vi "Sensors Begin.vi"   [LabVIEW 2013]
uses:
  <vilib>/Rock Robotics/SystemInterfaces/AI/FPGA_AIChannel.ctl
  <vilib>/Rock Robotics/SystemInterfaces/Typedef/FPGA_TypedefAnalogModule.ctl
types:
  T1 = typedef "FPGA_AIChannel.ctl" = enum8{"AI 1", "AI 2", "AI 3", "AI 4", "AI 5", "AI 6", "AI 7", "AI 8", "Invalid"}
  T2 = typedef "FPGA_TypedefAnalogModule.ctl" = enum16{"Analog Module 1", "Analog Module 2"}
  T3 = typedef "WPI_AnalogChannelDevRef.ctl" = cluster{"DevStatus":errorcluster, "Analog Module":T2, "Analog Channel":T1}
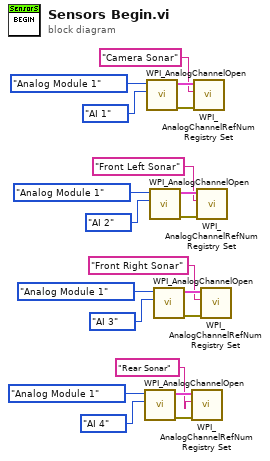
[diagram p0: block diagram]
diagram:
  n1 = call <vilib>:"WPI_AnalogChannelOpen.vi"("Analog Channel"=FPGA_AIChannel."AI 4", "Analog Module (Module 1)"=FPGA_TypedefAnalogModule."Analog Module 1") -> ("error out"=w5:errorcluster, "AIDeviceRef"=w4:T3)  [unwired: 8 in]
  n2 = call <vilib>:"WPI_AnalogChannelOpen.vi"("Analog Channel"=FPGA_AIChannel."AI 1", "Analog Module (Module 1)"=FPGA_TypedefAnalogModule."Analog Module 1") -> ("error out"=w19:errorcluster, "AIDeviceRef"=w20:T3)  [unwired: 8 in]
  n3 = call <vilib>:"WPI_AnalogChannelOpen.vi"("Analog Channel"=FPGA_AIChannel."AI 2", "Analog Module (Module 1)"=FPGA_TypedefAnalogModule."Analog Module 1") -> ("error out"=w13:errorcluster, "AIDeviceRef"=w12:T3)  [unwired: 8 in]
  n4 = call <vilib>:"WPI_AnalogChannelOpen.vi"("Analog Channel"=FPGA_AIChannel."AI 3", "Analog Module (Module 1)"=FPGA_TypedefAnalogModule."Analog Module 1") -> ("error out"=w10:errorcluster, "AIDeviceRef"=w11:T3)  [unwired: 8 in]
  n5 = call <vilib>:"WPI_AnalogChannelRefNum Registry Set.vi"("error in (no error)"=w5, "refnum name"="Rear Sonar", "AIDeviceRef"=w4) -> ()  [unwired: 7 in, 2 out]
  n6 = call <vilib>:"WPI_AnalogChannelRefNum Registry Set.vi"("error in (no error)"=w19, "refnum name"="Camera Sonar", "AIDeviceRef"=w20) -> ()  [unwired: 7 in, 2 out]
  n7 = call <vilib>:"WPI_AnalogChannelRefNum Registry Set.vi"("error in (no error)"=w13, "refnum name"="Front Left Sonar", "AIDeviceRef"=w12) -> ()  [unwired: 7 in, 2 out]
  n8 = call <vilib>:"WPI_AnalogChannelRefNum Registry Set.vi"("error in (no error)"=w10, "refnum name"="Front Right Sonar", "AIDeviceRef"=w11) -> ()  [unwired: 7 in, 2 out]
